vi "TDMS - File Viewer.vi"(8 "error in":errorcluster, 11 "file in":path) -> (0 "error out":errorcluster={"status"=TRUE, "code"=118, "source"="TDMS Open in TDMS - File Viewer with Flat Layout.vi"}, 3 "file out":path)   [LabVIEW 2020, in "TdmsFileViewer.lvlib"]
doc: "Opens the .tdms file specified in the <B>file path</B> input and presents the file data in the TDMS File Viewer dialog box."
uses:
  _TDMS File Viewer/TdmsFileViewer.lvlib
  <vilib>/Utility/error.llb/DialogType.ctl
  _TDMS File Viewer/Global VI for Localized Text.vi
panel:
  in  "File Tree":string[](tree)
  out "Property Table":string[][](table)
  in  "All":bool
  in  "Samples":i64=100000 min=-1 step=1
  in  "Start index":i64 min=0 step=1
  out "Waveform Graph":waveform(dbl)[](graph)
  in  "Value Table":i32(listbox)=-1
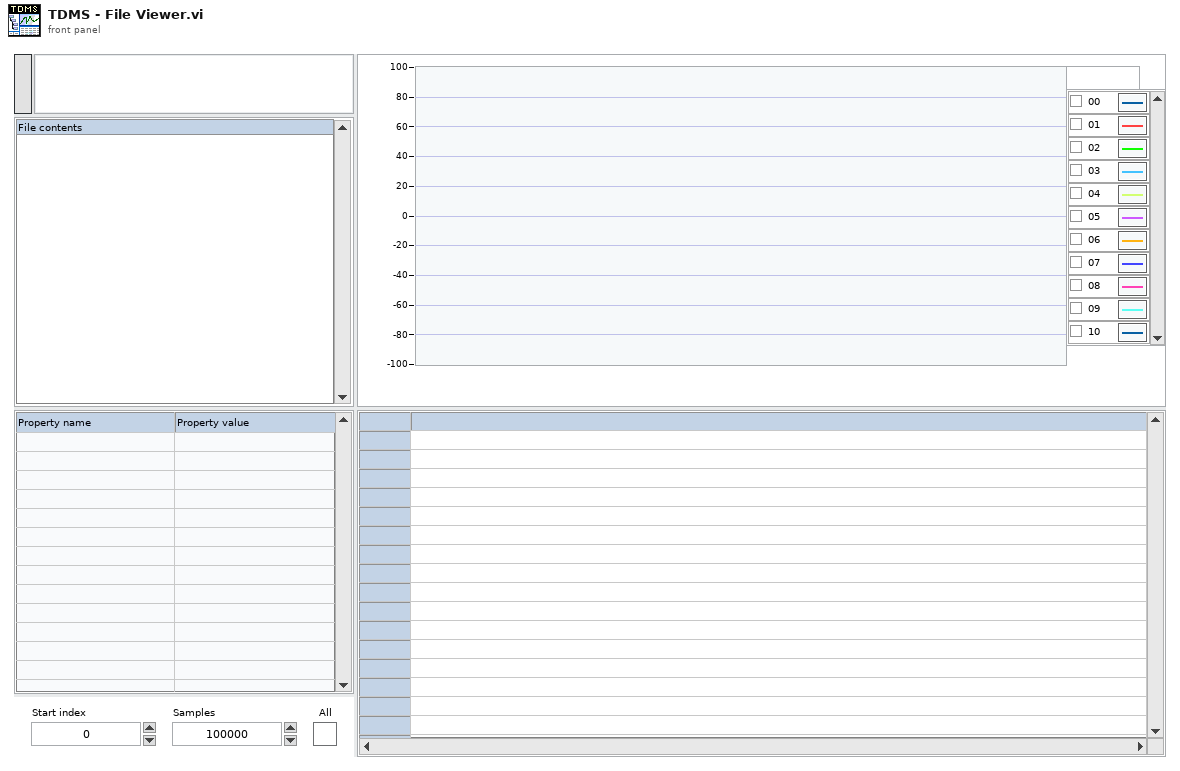
[diagram p1: front panel]
types:
  T1 = enum16{"open", "open or create", "create or replace", "create", "open (read-only)"}
  T2 = cluster{"All":bool, "Start index":i64, "Samples":i64}
  T3 = enum8{"Enabled", "Disabled", "Disabled and Grayed Out"}
  T4 = typedef "eventvkey.ctl" = enum16{"ASCII", "Enter", "Return", "Shift", "Ctrl", "Alt", "Cmd", "Opt", "Caps", "NumLock", "Clear", "Break", "Up", "Down", "Left", "Right", "Insert", "Delete", "Home", "End", "PageUp", "PageDown", "Escape", "Help", "Pause", "ScrollLock", "F1", "F2", "F3", "F4", "F5", "F6", "F7", "F8", "F9", "F10", "F11", "F12", "F13", "F14", "F15", "F16", "F17", "F18", "F19", "F20", "F21", "F22", "F23", "F24", "Play", "VolumeUp", "VolumeDown", "Mute", "Two Byte Char"}
  T5 = typedef "LVPoint32TypeDef.ctl" = cluster{"Horizontal":i32, "Vertical":i32}
  T6 = typedef "TdmsFileViewer.lvlib/Table Components.ctl" = cluster{"column headers":string[], "row headers":string[], "values":string[][]}
  T7 = typedef "DialogType.ctl" = u16
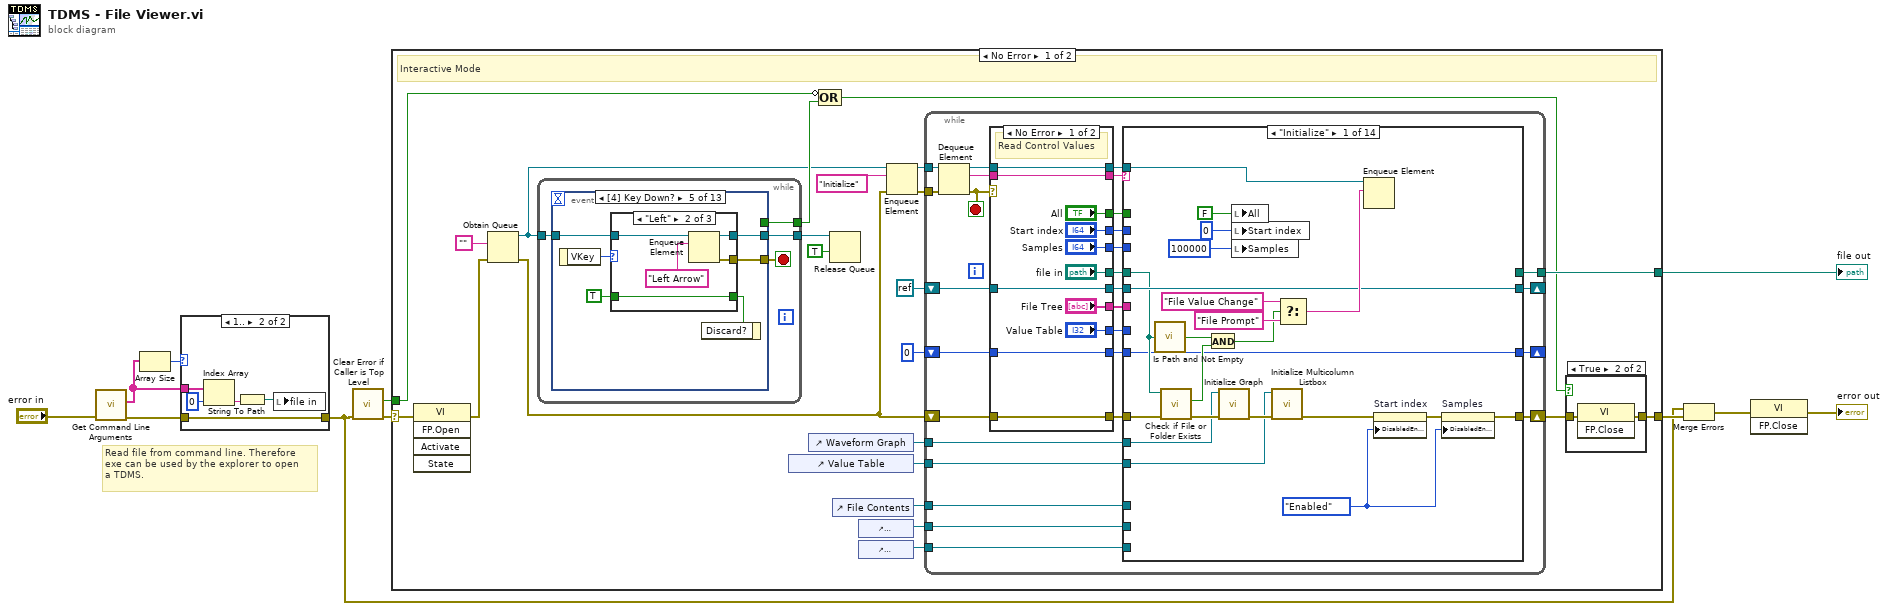
[diagram p0: block diagram]
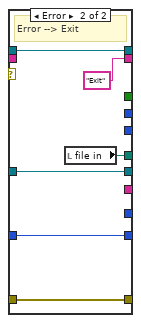
[diagram p4: hidden frame]
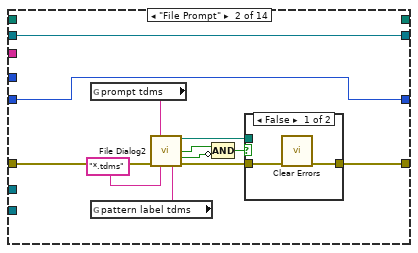
[diagram p5: hidden frame]
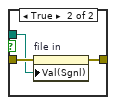
[diagram p6: hidden frame]
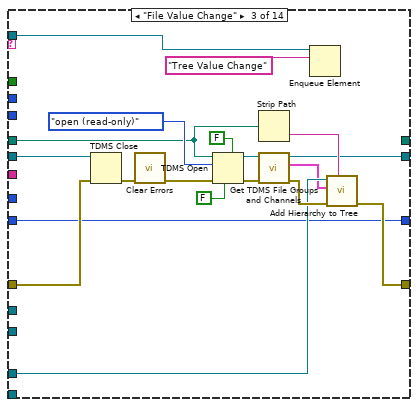
[diagram p7: hidden frame]
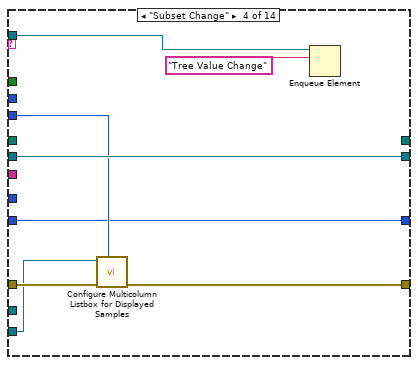
[diagram p8: hidden frame]
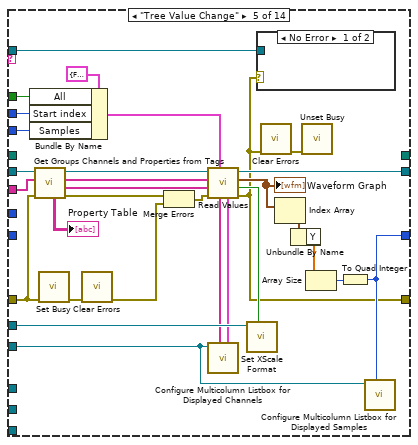
[diagram p9: hidden frame]
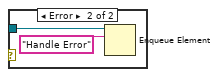
[diagram p10: hidden frame]
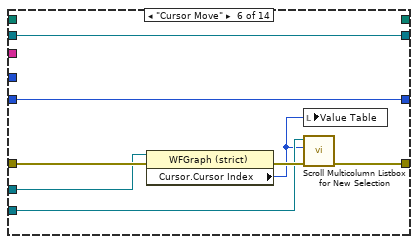
[diagram p11: hidden frame]
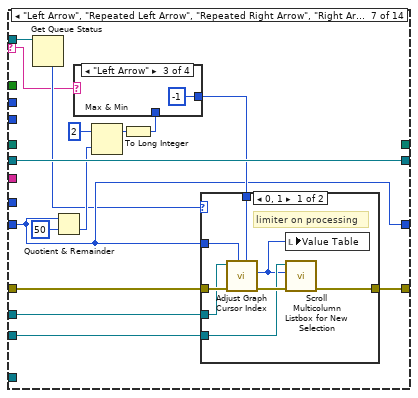
[diagram p12: hidden frame]
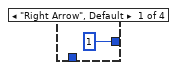
[diagram p14: hidden frame]
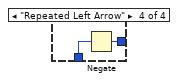
[diagram p16: hidden frame]
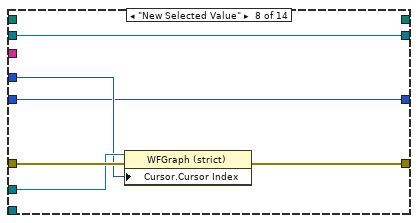
[diagram p17: hidden frame]
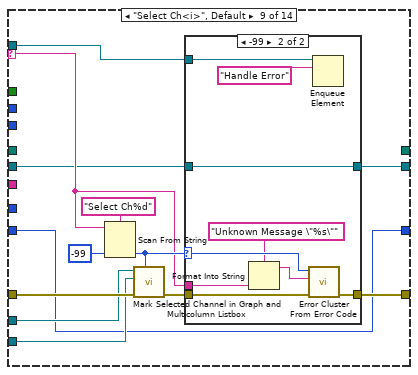
[diagram p18: hidden frame]
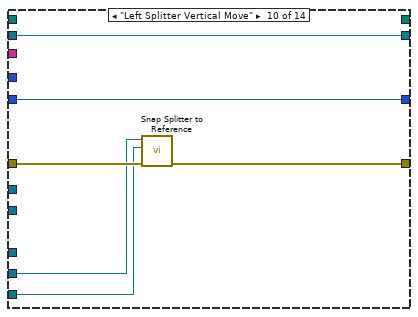
[diagram p20: hidden frame]
diagram:
  # "Read file from command line. Therefore\nexe can be used by the explorer to open\na TDMS."
  n1 = call <vilib>:"Get Command Line Arguments.vi"("error in (no error)"="error in") -> ("error out"=w3:errorcluster, "arguments"=w4:string[])  [unwired: 8 in, 1 out]
  n2 = Array Size(array=w4) -> (size(s)=w1:i32)
  n3 = case shown="1.." w1 {
    tunnel: w4 -> [_ w17]
    tunnel: w3 -> [w12 w13]
    tunnel: [w12 w13] -> w2
    frame Default {
    }
    frame 1.. {
      n4 = Index Array(array=w17, index=0) -> (element=w15:string)
      n5 = String To Path(string=w15) -> (path=w14:path)
      n6 = local write "file in"(w14) -> ()
    }
  }
  n7 = call "Clear Error if Caller is Top Level.vi"("error in"=w2) -> ("error out"=w11:errorcluster, "top level"=w8:bool)  [unwired: 9 in]
  n8 = case shown="No Error" w11 {
    selector: w11 -> [w20 w398]
    tunnel: [w31 _] -> w9
    tunnel: [w39 w398] -> w10
    tunnel: w8 -> [w27 _]
    frame No Error {
      # "Interactive Mode"
      n9 = invoke class="VI" method="FP.Open"(error in=w20) -> (error out=w19:errorcluster)  [unwired: 4 in, 4 out]
      n10 = Obtain Queue(element data type="", error in (no error)=w19) -> (queue out=w18:refnum<queue>, error out=w21:errorcluster)  [unwired: 3 in, 1 out]
      n11 = while {
        tunnel: [w292] -> w30
        tunnel: w18 -> [w291]
        tunnel: [w290] -> w25
        stop <- w293 stop-if-true
        n12 = event shown="[4] Key Down?" {
          selector: _ -> [_ _ _ _ _ _ _ _ _ _ _ _ _]
          dyn-events: _ -> [_ _ _ _ _ _ _ _ _ _ _ _ _]
          timeout: _ -> [_ _ _ _ _ _ _ _ _ _ _ _ _]
          tunnel: [w295 w304 w312 w327 w331 w348 w365 w369 w373 w382 w386 w390 w394] -> w293
          tunnel: [_ _ _ _ _ _ _ _ _ _ _ _ w396] -> w292
          tunnel: w291 -> [w296 w305 w313 w328 w332 w349 w366 w370 w374 w383 w387 w391 w395]
          tunnel: [w294 w303 w311 w326 w330 w347 w364 w368 w372 w381 w385 w389 w393] -> w290
          event "Start index", "Samples": Value Change {
            n13 = event-data() -> ()  [unwired: 1 in, 1 out]
            n14 = local read "Start index"() -> (w301:i64)
            n15 = local read "Samples"() -> (w300:i64)
            n16 = Less Than 0?(x=w300) -> (x < 0?=w299:bool)
            n17 = Equal To 0?(x=w301) -> (x = 0?=w298:bool)
            n18 = And(x=w299, y=w298) -> (x .and. y?=w297:bool)
            n19 = local write "All"(w297) -> ()
            n20 = Enqueue Element(queue=w296, element="Subset Change" ("CHM or HLP filename (lvdialog.chm)")) -> (queue out=w294:refnum<queue>, error out=w295:errorcluster)  [unwired: 2 in, 1 out]
          }
          event "All": Value Change {
            n21 = event-data() -> ("NewVal"=w307:bool)  [unwired: 1 in]
            n22 = Select(t=T3."Disabled and Grayed Out" ("Disabled"), s=w307, f=T3."Enabled" ("Disabled")) -> (s? t:f=w306:T3)
            n23 = property on="Start index" class="DigNum (strict)"("DisabledEnum"=w306) -> ()  [unwired: 2 in, 2 out]
            n24 = property on="Samples" class="DigNum (strict)"("DisabledEnum"=w306) -> ()  [unwired: 2 in, 2 out]
            n25 = Enqueue Element(queue=w305, element="Subset Change" ("CHM or HLP filename (lvdialog.chm)")) -> (queue out=w303:refnum<queue>, error out=w304:errorcluster)  [unwired: 2 in, 1 out]
          }
          event "file in": Value Change {
            n26 = event-data() -> ("OldVal"=w314:path, "NewVal"=w318:path)  [unwired: 1 in]
            n27 = call <vilib>:"Is Path and Not Empty.vi"("path"=w318) -> ("Is Path and Not Empty?"=w317:bool)  [unwired: 4 in]
            n28 = call <vilib>:"Check if File or Folder Exists.vi"("path"=w318) -> ("file or folder exists?"=w316:bool)  [unwired: 8 in, 2 out]
            n29 = And(x=w316, y=w317) -> (x .and. y?=w315:bool)
            n30 = case shown="False" w315 {
              tunnel: "File Value Change" ("CHM or HLP filename (lvdialog.chm)") -> [_ w325]
              tunnel: w314 -> [w321 _]
              tunnel: w313 -> [w320 w324]
              tunnel: [_ w323] -> w312
              tunnel: [w320 w322] -> w311
              frame False {
                n31 = local write "file in"(w321) -> ()
              }
              frame True {
                n32 = Enqueue Element(queue=w324, element=w325) -> (queue out=w322:refnum<queue>, error out=w323:errorcluster)  [unwired: 2 in, 1 out]
              }
            }
          }
          event "File Tree": Value Change {
            n33 = event-data() -> ()  [unwired: 1 in, 1 out]
            n34 = Enqueue Element(queue=w328, element="Tree Value Change" ("CHM or HLP filename (lvdialog.chm)")) -> (queue out=w326:refnum<queue>, error out=w327:errorcluster)  [unwired: 2 in, 1 out]
          }
          event Key Down? {
            n35 = event-data() -> ("VKey"=w335:T4)  [unwired: 1 in]
            n36 = case shown="\"Left\"" w335 {
              tunnel: [_ w340 w345] -> w333
              tunnel: TRUE ("Discard?") -> [_ w340 w345]
              tunnel: w332 -> [w336 w339 w344]
              tunnel: [_ w338 w343] -> w331
              tunnel: [w336 w337 w342] -> w330
              frame Default {
              }
              frame "Left" {
                n37 = Enqueue Element(queue=w339, element="Left Arrow" ("CHM or HLP filename (lvdialog.chm)")) -> (queue out=w337:refnum<queue>, error out=w338:errorcluster)  [unwired: 2 in, 1 out]
              }
              frame "Right" {
                n38 = Enqueue Element(queue=w344, element="Right Arrow" ("CHM or HLP filename (lvdialog.chm)")) -> (queue out=w342:refnum<queue>, error out=w343:errorcluster)  [unwired: 2 in, 1 out]
              }
            }
            n39 = event-data("Discard?"=w333) -> ()  [unwired: 1 in, 1 out]
          }
          event event type 5.0.x8000000b {
            n40 = event-data() -> ("VKey"=w352:T4)  [unwired: 1 in]
            n41 = case shown="\"Right\"" w352 {
              tunnel: [_ w357 w362] -> w351
              tunnel: TRUE ("abort (F)") -> [_ w357 w362]
              tunnel: w349 -> [w353 w356 w361]
              tunnel: [_ w355 w360] -> w348
              tunnel: [w353 w354 w359] -> w347
              frame Default {
              }
              frame "Left" {
                n42 = Enqueue Element(queue=w356, element="Repeated Left Arrow" ("CHM or HLP filename (lvdialog.chm)")) -> (queue out=w354:refnum<queue>, error out=w355:errorcluster)  [unwired: 2 in, 1 out]
              }
              frame "Right" {
                n43 = Enqueue Element(queue=w361, element="Repeated Right Arrow" ("CHM or HLP filename (lvdialog.chm)")) -> (queue out=w359:refnum<queue>, error out=w360:errorcluster)  [unwired: 2 in, 1 out]
              }
            }
            n44 = event-data("Discard?"=w351) -> ()  [unwired: 1 in, 1 out]
          }
          event "Waveform Graph": Cursor Move {
            n45 = event-data() -> ()  [unwired: 1 in, 1 out]
            n46 = Enqueue Element(queue=w366, element="Cursor Move" ("CHM or HLP filename (lvdialog.chm)")) -> (queue out=w364:refnum<queue>, error out=w365:errorcluster)  [unwired: 2 in, 1 out]
          }
          event "Value Table": Value Change {
            n47 = event-data() -> ()  [unwired: 1 in, 1 out]
            n48 = Enqueue Element(queue=w370, element="New Selected Value" ("CHM or HLP filename (lvdialog.chm)")) -> (queue out=w368:refnum<queue>, error out=w369:errorcluster)  [unwired: 2 in, 1 out]
          }
          event "Value Table": Double Click {
            n49 = event-data() -> ("CtlRef"=w380:refnum<vi>, "Coords"=w375:T5)  [unwired: 1 in]
            n50 = call "Coordinates to Multicolumn Listbox Column.vi"("Coords"=w375, "MulticolumnListbox in"=w380) -> ("Column"=w378:i32)  [unwired: 9 in]
            n51 = Format Into String(format string="%d", initial string="Select Ch" ("CHM or HLP filename (lvdialog.chm)"), w378) -> (resulting string=w376:string)  [unwired: 1 in, 1 out]
            n52 = Enqueue Element(queue=w374, element=w376) -> (queue out=w372:refnum<queue>, error out=w373:errorcluster)  [unwired: 2 in, 1 out]
          }
          event Mouse Leave; Mouse Up {
            n53 = event-data() -> ()  [unwired: 1 in, 1 out]
            n54 = Enqueue Element(queue=w383, element="Left Splitter Vertical Move" ("CHM or HLP filename (lvdialog.chm)")) -> (queue out=w381:refnum<queue>, error out=w382:errorcluster)  [unwired: 2 in, 1 out]
          }
          event Mouse Leave; Mouse Up {
            n55 = event-data() -> ()  [unwired: 1 in, 1 out]
            n56 = Enqueue Element(queue=w387, element="Right Splitter Vertical Move" ("CHM or HLP filename (lvdialog.chm)")) -> (queue out=w385:refnum<queue>, error out=w386:errorcluster)  [unwired: 2 in, 1 out]
          }
          event Pane Size {
            n57 = event-data() -> ()  [unwired: 1 in, 1 out]
            n58 = Enqueue Element(queue=w391, element="Graph Resize" ("CHM or HLP filename (lvdialog.chm)")) -> (queue out=w389:refnum<queue>, error out=w390:errorcluster)  [unwired: 2 in, 1 out]
          }
          event Panel Close? {
            w394 = errorcluster {"status"=TRUE, "code"=0, "source"=""}  # Stop
            w396 = TRUE ("Discard?")
            n59 = event-data() -> ()  [unwired: 1 in, 1 out]
            n60 = Enqueue Element(queue=w395, element="Exit" ("CHM or HLP filename (lvdialog.chm)")) -> (queue out=w393:refnum<queue>)  [unwired: 2 in, 2 out]
            n61 = event-data("Discard?"=w396) -> ()  [unwired: 1 in, 1 out]
          }
        }
      }
      n62 = control-ref of="Value Table"() -> (w37:refnum<vi>)
      n63 = control-ref of="Waveform Graph"() -> (w34:refnum<vi>)
      n64 = Compound Arithmetic op=OR(invert w27, w30) -> (w29:bool)
      n65 = Release Queue(queue=w25, force destroy? (F)=TRUE) -> ()  [unwired: 1 in, 3 out]
      n66 = control-ref of="File Contents"() -> (w36:refnum<vi>)
      n67 = control-ref of="Splitter:ValueTableTop"() -> (w33:refnum<vi>)
      n68 = control-ref of="Splitter:PropTableTop"() -> (w32:refnum<vi>)
      n69 = Enqueue Element(queue=w18, element="Initialize" ("CHM or HLP filename (lvdialog.chm)"), error in (no error)=w21) -> (queue out=w26:refnum<queue>, error out=w23:errorcluster)  [unwired: 1 in, 1 out]
      n70 = while {
        tunnel: w26 -> [w68]
        shift-right: [w57] -> _
        shift-left: refnum<k0> refnum -> [w58]
        shift-right: [w69] -> w40
        shift-left: w21 -> [w70]
        tunnel: w37 -> [w56]
        tunnel: w36 -> [w55]
        tunnel: w34 -> [w53]
        tunnel: w33 -> [w52]
        tunnel: w32 -> [w51]
        tunnel: [w50] -> w31
        shift-right: [w47] -> _
        shift-left: i64 0 -> [w48]
        tunnel: w23 -> [w44]
        stop <- w67 stop-if-true
        n71 = Dequeue Element(queue=w68, error in (no error)=w44) -> (queue out=w46:refnum<queue>, element=w65:string, error out=w67:errorcluster)  [unwired: 1 in, 1 out]
        n72 = case shown="No Error" w67 {
          tunnel: [w81 "Exit" ("element")] -> w66
          tunnel: w65 -> [w81 _]
          tunnel: ["file in" w85] -> w64
          tunnel: ["File Tree" _] -> w63
          tunnel: ["Samples" _] -> w62
          tunnel: ["Start index" _] -> w61
          tunnel: ["All" _] -> w60
          tunnel: [w75 w86] -> w59
          tunnel: w58 -> [w75 w86]
          tunnel: [w82 w88] -> w71
          tunnel: w70 -> [w82 w88]
          tunnel: ["Value Table" _] -> w54
          tunnel: [w73 w84] -> w49
          tunnel: w48 -> [w73 w84]
          tunnel: [w72 w83] -> w45
          tunnel: w46 -> [w72 w83]
          frame No Error {
            # "Read Control Values"
          }
          frame Error {
            # "Error --> Exit"
            n73 = local read "file in"() -> (w85:path)
          }
        }
        n74 = case shown="\"Initialize\"" w66 {
          selector: w66 -> [_ _ _ _ _ _ w195 _ w233 _ _ _ _ _]
          tunnel: w64 -> [w104 _ w129 _ _ _ _ _ _ _ _ _ _ w286]
          tunnel: w63 -> [_ _ _ _ w163 _ _ _ _ _ _ _ _ _]
          tunnel: w62 -> [_ _ _ w149 w176 _ _ _ _ _ _ _ _ _]
          tunnel: w61 -> [_ _ _ _ w177 _ _ _ _ _ _ _ _ _]
          tunnel: w60 -> [_ _ _ _ w178 _ _ _ _ _ _ _ _ _]
          tunnel: w56 -> [w91 _ _ w150 w166 w189 w205 _ w236 _ _ _ _ _]
          tunnel: w59 -> [w105 w114 w135 w152 w180 w191 w207 w227 w230 w257 w263 w270 w275 w288]
          tunnel: [w105 w114 w131 w152 w179 w191 w207 w227 w231 w257 w263 w270 w275 refnum<k0> refnum] -> w57
          tunnel: w71 -> [w110 w122 w145 w154 w161 w194 w209 w228 w242 w259 w264 w273 w277 w289]
          tunnel: w55 -> [_ _ w134 _ _ _ _ _ _ _ _ _ _ _]
          tunnel: [w107 w120 w141 w153 w162 w192 w208 w229 w240 w258 w265 w271 w276 w289] -> w69
          tunnel: w54 -> [_ _ _ _ _ _ _ w225 _ _ _ _ _ _]
          tunnel: w53 -> [w103 _ _ _ w174 w190 w206 w226 w237 _ _ w269 _ _]
          tunnel: w52 -> [_ _ _ _ _ _ _ _ _ w256 w262 w268 _ _]
          tunnel: w51 -> [_ _ _ _ _ _ _ _ _ w255 w261 w267 _ _]
          tunnel: [_ _ _ _ _ _ _ _ _ _ _ _ _ w286] -> w50
          tunnel: w49 -> [w93 w111 w130 w148 _ w187 w203 w224 w234 w254 w260 w266 w274 w285]
          tunnel: [w93 w111 w130 w148 w165 w187 w203 w224 w234 w254 w260 w266 w274 w285] -> w47
          tunnel: w45 -> [w90 _ w128 w147 w155 _ w197 _ w232 _ _ _ _ _]
          frame "Initialize" {
            w94 = T3."Enabled" ("Disabled")
            n75 = call <vilib>:"Is Path and Not Empty.vi"("path"=w104) -> ("Is Path and Not Empty?"=w100:bool)  [unwired: 4 in]
            n76 = call <vilib>:"Check if File or Folder Exists.vi"("error in (no error)"=w110, "path"=w104) -> ("error out"=w109:errorcluster, "file or folder exists?"=w99:bool)  [unwired: 7 in, 1 out]
            n77 = And(x=w100, y=w99) -> (x .and. y?=w98:bool)
            n78 = call "Initialize Graph.vi"("error in"=w109, "WaveformGraph"=w103) -> ("error out"=w92:errorcluster)  [unwired: 9 in]
            n79 = local write "All"(FALSE ("All")) -> ()
            n80 = local write "Start index"(i64 0 ("Start index")) -> ()
            n81 = local write "Samples"(i64 100000 ("Samples")) -> ()
            n82 = call "Initialize Multicolumn Listbox.vi"("error in"=w92, "MulticolumnListbox"=w91) -> ("error out"=w89:errorcluster)  [unwired: 9 in]
            n83 = Select(t="File Value Change" ("CHM or HLP filename (lvdialog.chm)"), s=w98, f="File Prompt" ("CHM or HLP filename (lvdialog.chm)")) -> (s? t:f=w106:string)
            n84 = Enqueue Element(queue=w90, element=w106) -> ()  [unwired: 2 in, 3 out]
            n85 = property on="Start index" class="DigNum (strict)"(error in=w89, "DisabledEnum"=w94) -> (error out=w108:errorcluster)  [unwired: 1 in, 1 out]
            n86 = property on="Samples" class="DigNum (strict)"(error in=w108, "DisabledEnum"=w94) -> (error out=w107:errorcluster)  [unwired: 1 in, 1 out]
          }
          frame "File Prompt" {
            n87 = global read "Global VI for Localized Text.vi" "prompt tdms"() -> (w118:string)
            n88 = global read "Global VI for Localized Text.vi" "pattern label tdms"() -> (w117:string)
            n89 = call "File Dialog2"("prompt"=w118, "error in"=w122, "pattern (all files)"="*.tdms", "pattern label"=w117) -> ("selected path"=w115:path, "exists"=w113:bool, "cancelled"=w112:bool, "error out"=w121:errorcluster)  [unwired: 3 in, 5 out]
            n90 = Compound Arithmetic op=AND(w113, invert w112) -> (w116:bool)
            n91 = case shown="False" w116 {
              tunnel: w121 -> [w124 w127]
              tunnel: [w123 w126] -> w120
              tunnel: w115 -> [_ w125]
              frame False {
                n92 = call <vilib>:"Clear Errors.vi"("error in (no error)"=w124) -> ("error out"=w123:errorcluster)  [unwired: 5 in, 1 out]
              }
              frame True {
                n93 = property on="file in" class="Path"(error in=w127, "Val(Sgnl)"=w125) -> (error out=w126:errorcluster)  [unwired: 1 in, 1 out]
              }
            }
          }
          frame "File Value Change" {
            n94 = TDMS Close(8:w145, 11:w135) -> (0:w144:errorcluster)  [unwired: 1 out]
            n95 = call <vilib>:"Clear Errors.vi"("error in (no error)"=w144) -> ("error out"=w143:errorcluster)  [unwired: 5 in, 1 out]
            n96 = TDMS Open(5:FALSE ("create index file? (T)"), 6:FALSE ("disable buffering (T)"), 8:w143, 10:T1."open (read-only)" ("operation"), 11:w129) -> (0:w146:errorcluster, 3:w136:refnum<k34>)  [unwired: 2 in]
            n97 = Strip Path(path=w129) -> (name=w133:string)  [unwired: 1 out]
            n98 = call "Get TDMS File Groups and Channels.vi"("error in"=w146, "TDMS ref in"=w136) -> ("error out"=w142:errorcluster, "file contents"=w132:cluster{string, string[]}[], "TDMS ref out"=w131:refnum<k34>)  [unwired: 7 in]
            n99 = Enqueue Element(queue=w128, element="Tree Value Change" ("CHM or HLP filename (lvdialog.chm)")) -> ()  [unwired: 2 in, 3 out]
            n100 = call "Add Hierarchy to Tree.vi"("file name"=w133, "error in"=w142, "file contents"=w132, "file tree refnum"=w134) -> ("error out"=w141:errorcluster)  [unwired: 7 in]
          }
          frame "Subset Change" {
            n101 = call "Configure Multicolumn Listbox for Displayed Samples.vi"("Samples"=w149, "error in"=w154, "MulticolumnListbox in"=w150) -> ("error out"=w153:errorcluster)  [unwired: 7 in, 1 out]
            n102 = Enqueue Element(queue=w147, element="Tree Value Change") -> ()  [unwired: 2 in, 3 out]
          }
          frame "Tree Value Change" {
            n103 = Bundle By Name(cluster=T2 {"All"=FALSE, "Start index"=0, "Samples"=0}, "All"=w178, "Start index"=w177, "Samples"=w176) -> (w175:T2)
            n104 = call "Get Groups Channels and Properties from Tags.vi"("error in"=w161, "File Tree"=w163, "tdms file in"=w180) -> ("error out"=w158:errorcluster, "channel names out"=w183:string[], "group names out"=w182:string[], "tdms file out"=w181:refnum<k34>, "property table"=→"Property Table":string[][])  [unwired: 2 in]
            n105 = call <vilib>:"Set Busy.vi"("error in (no error)"=w161) -> ("error out"=w164:errorcluster)  [unwired: 9 in, 1 out]
            n106 = call <vilib>:"Clear Errors.vi"("error in (no error)"=w164) -> ("error out"=w160:errorcluster)  [unwired: 5 in, 1 out]
            n107 = Merge Errors(w158, w160) -> (w159:errorcluster)
            n108 = call "Read Values.vi"("read subset"=w175, "error in"=w159, "channel names"=w183, "group names"=w182, "tdms file"=w181) -> ("error out"=w162:errorcluster, "waveform timestamps = 0"=w169:bool, "waveform values"=w170:waveform(dbl)[], "tdms file out"=w179:refnum<k34>, "table values"=w173:T6, "widest value strings"=w171:string[])  [unwired: 1 in]
            "Waveform Graph" <- w170
            n109 = call "Configure Multicolumn Listbox for Displayed Channels.vi"("table values"=w173, "widest value strings"=w171, "MulticolumnListbox in"=w166) -> ()  [unwired: 7 in]
            n110 = call "Set XScale Format.vi"("timestamp eq 0"=w169, "Waveform Graph"=w174) -> ()  [unwired: 8 in]
            n111 = case shown="No Error" w162 {
              tunnel: w155 -> [_ w185]
              frame No Error {
              }
              frame Error {
                n112 = Enqueue Element(queue=w185, element="Handle Error") -> ()  [unwired: 2 in, 3 out]
              }
            }
            n113 = call <vilib>:"Clear Errors.vi"("error in (no error)"=w162) -> ("error out"=w184:errorcluster)  [unwired: 5 in, 1 out]
            n114 = Index Array(array=w170) -> (element=w167:waveform(dbl))  [unwired: 1 in]
            n115 = Unbundle By Name(w167) -> ("Y"=w168:dbl[])
            n116 = call <vilib>:"Unset Busy.vi"("error in (no error)"=w184) -> ()  [unwired: 10 in, 1 out]
            n117 = Array Size(array=w168) -> (size(s)=w157:i32)
            n118 = To Quad Integer(1:w157) -> (0:w165:i64)
            n119 = call "Configure Multicolumn Listbox for Displayed Samples.vi"("Samples"=w165, "MulticolumnListbox in"=w166) -> ()  [unwired: 8 in, 2 out]
          }
          frame "Cursor Move" {
            n120 = property class="WFGraph (strict)"(reference=w190, error in=w194) -> (error out=w193:errorcluster, "Cursor.Cursor Index"=w188:i32)  [unwired: 1 out]
            n121 = local write "Value Table"(w188) -> ()
            n122 = call "Scroll Multicolumn Listbox for New Selection.vi"("error in"=w193, "new index"=w188, "MulticolumnListbox"=w189) -> ("error out"=w192:errorcluster)  [unwired: 8 in]
          }
          frame "Left Arrow", "Repeated Left Arrow", "Repeated Right Arrow", "Right Arrow" {
            n123 = Get Queue Status(queue=w197) -> (# elements in queue=w196:i32)  [unwired: 2 in, 7 out]
            n124 = Quotient & Remainder(x=w203, y=i64 50) -> (floor(x/y)=w201:i64)  [unwired: 1 out]
            n125 = Max & Min(x=i64 2, y=w201) -> (max(x,y)=w199:i64)  [unwired: 1 out]
            n126 = To Long Integer(number=w199) -> (32bit integer=w198:i32)
            n127 = case shown="\"Left Arrow\"" w195 {
              tunnel: [1 w220 -1 w222] -> w204
              tunnel: w198 -> [_ w220 _ w223]
              frame "Right Arrow", Default {
              }
              frame "Repeated Right Arrow" {
              }
              frame "Left Arrow" {
              }
              frame "Repeated Left Arrow" {
                n128 = Negate(x=w223) -> (-x=w222:i32)
              }
            }
            n129 = case shown="0, 1" w196 {
              tunnel: w206 -> [w214 _]
              tunnel: w209 -> [w217 w218]
              tunnel: w205 -> [w213 _]
              tunnel: [w215 w218] -> w208
              tunnel: w204 -> [w211 _]
              tunnel: w203 -> [w210 _]
              frame 0, 1 {
                # "limiter on processing"
                n130 = call "Adjust Graph Cursor Index.vi"("index adjustment"=w211, "Plot 0 samples"=w210, "error in"=w217, "WaveformGraph in"=w214) -> ("error out"=w216:errorcluster, "adjusted index"=w212:i32)  [unwired: 6 in]
                n131 = local write "Value Table"(w212) -> ()
                n132 = call "Scroll Multicolumn Listbox for New Selection.vi"("error in"=w216, "new index"=w212, "MulticolumnListbox"=w213) -> ("error out"=w215:errorcluster)  [unwired: 8 in]
              }
              frame Default {
                # "When message backlog is high, we don't execute time consuming code to adjust graph cursor position and value table"
              }
            }
          }
          frame "New Selected Value" {
            n133 = property class="WFGraph (strict)"(reference=w226, error in=w228, "Cursor.Cursor Index"=w225) -> (error out=w229:errorcluster)  [unwired: 1 out]
          }
          frame "Select Ch<i>", Default {
            n134 = Scan From String(format string="Select Ch%d", input string=w233, default 1=-99 ("default value 1")) -> (output 1=w235:i32)  [unwired: 2 in, 3 out]
            n135 = call "Mark Selected Channel in Graph and Multicolumn Listbox.vi"("selected channel"=w235, "error in"=w242, "Value Table"=w236, "WaveformGraph"=w237) -> ("error out"=w241:errorcluster)  [unwired: 7 in]
            n136 = case shown="-99" w235 {
              selector: w235 -> [_ w251]
              tunnel: w241 -> [w244 w253]
              tunnel: [w244 w252] -> w240
              tunnel: w233 -> [_ w249]
              tunnel: w232 -> [_ w246]
              tunnel: [w243 w245] -> w231
              tunnel: w230 -> [w243 w245]
              frame Default {
              }
              frame -99 {
                n137 = Format Into String(format string="Unknown Message \"%s\"", w249) -> (resulting string=w248:string)  [unwired: 2 in, 1 out]
                n138 = call <vilib>:"Error Cluster From Error Code.vi"("error in (no error)"=w253, "error message (\"\")"=w248, "error code (0)"=w251) -> ("error out"=w252:errorcluster)  [unwired: 6 in]
                n139 = Enqueue Element(queue=w246, element="Handle Error") -> ()  [unwired: 2 in, 3 out]
              }
            }
          }
          frame "Left Splitter Vertical Move" {
            n140 = call "Snap Splitter to Reference.vi"("error in"=w259, "splitter on move"=w255, "reference splitter"=w256) -> ("error out"=w258:errorcluster)  [unwired: 8 in]
          }
          frame "Right Splitter Vertical Move" {
            n141 = call "Snap Splitter to Reference.vi"("error in"=w264, "splitter on move"=w262, "reference splitter"=w261) -> ("error out"=w265:errorcluster)  [unwired: 8 in]
          }
          frame "Graph Resize" {
            n142 = call "Set Waveform Graph LegNumRows.vi"("error in"=w273, "WaveformGraph"=w269) -> ("error out"=w272:errorcluster)  [unwired: 9 in]
            n143 = call "Snap Splitter to Reference.vi"("error in"=w272, "splitter on move"=w267, "reference splitter"=w268) -> ("error out"=w271:errorcluster)  [unwired: 8 in]
          }
          frame "Handle Error" {
            n144 = case shown="Error .." w277 {
              selector: w277 -> [w278 w283]
              tunnel: [w278 w282] -> w276
              frame No Error {
                # "No Trouble Found"
              }
              frame Error {
                w281 = T7 4 items=["no dialog", "OK message", "continue or stop message", "OK message + warnings", "continue/stop + warnings"] ("type of dialog (OK msg:1)")
                # "Report errors"
                n145 = Unbundle By Name(w283) -> ("code"=w280:i32, "source"=w279:string)
                n146 = call <vilib>:"Simple Error Handler.vi"("error code (no error:0)"=w280, "error source (\" \")"=w279, "type of dialog (OK msg:1)"=w281, "error in (no error)"=w283) -> ("error out"=w284:errorcluster)  [unwired: 1 in, 4 out]
                n147 = call <vilib>:"Clear Errors.vi"("error in (no error)"=w284) -> ("error out"=w282:errorcluster)  [unwired: 5 in, 1 out]
              }
            }
          }
          frame "", "Exit" {
            n148 = TDMS Close(8:w289, 11:w288) -> ()  [unwired: 2 out]
          }
        }
      }
      n149 = case shown="True" w29 {
        tunnel: w40 -> [w41 w43]
        tunnel: [w41 w42] -> w39
        frame False {
        }
        frame True {
          n150 = invoke class="VI" method="FP.Close"(error in=w43) -> (error out=w42:errorcluster)  [unwired: 2 in, 2 out]
        }
      }
    }
    frame Error {
      # "If TDMS File Viewer running as subVI, input error immediately returns."
    }
  }
  "file out" <- w9
  n151 = Merge Errors(w2, w10) -> (w7:errorcluster)
  n152 = invoke class="VI" method="FP.Close"(error in=w7) -> (error out=→"error out":errorcluster)  [unwired: 2 in, 2 out]
